vi "Stop Core.vi"(10 "final error code":i32, 11 "Broadcast Actor in":refnum<class "Broadcast Actor.lvclass">) -> (3 "Broadcast Actor out":refnum<class "Broadcast Actor.lvclass">)   [LabVIEW 2017, in "Broadcast Actor.lvlib" / "Broadcast Actor.lvclass"]
doc: "(<B>Filename</B>: Actor Framework.lvlib:Actor.lvclass:Stop Core.vi)\n\nDefines what the actor does before it stops. Use the <B>final error code</B> input to determine whether the actor shut down in response to an error.\n\nBy default, this method does nothing. A descendant class may override it to define behavior, such as shutting down any processes the actor initiated in its override of the Actor Core method."
uses:
  Broadcast Actor.lvclass
  Broadcast Actor.lvclass/Broadcast Actor.ctl
  <vilib>/ActorFramework/Actor/Actor.lvclass
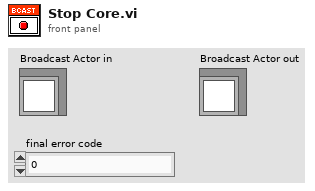
[diagram p1: front panel]
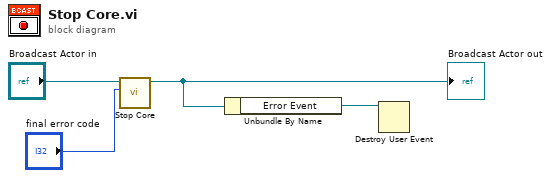
[diagram p0: block diagram]
diagram:
  n1 = call-parent "Stop Core.vi"("final error code"="final error code", "Actor in"="Broadcast Actor in") -> ("Actor out"=w2:refnum<class "Broadcast Actor.lvclass">)  [unwired: 9 in]
  "Broadcast Actor out" <- w2
  n2 = Unbundle By Name(w2) -> ("Error Event"=w1:refnum<user-event>)
  n3 = Destroy User Event(user event=w1) -> ()  [unwired: 1 in, 1 out]
